vi "_script_update_doc_txt_stub.vi"() -> ()   [LabVIEW 2014]
uses:
  JKI State Machine++.lvlib
panel:
  out "States":string
  out "appended array":path[](array[path])
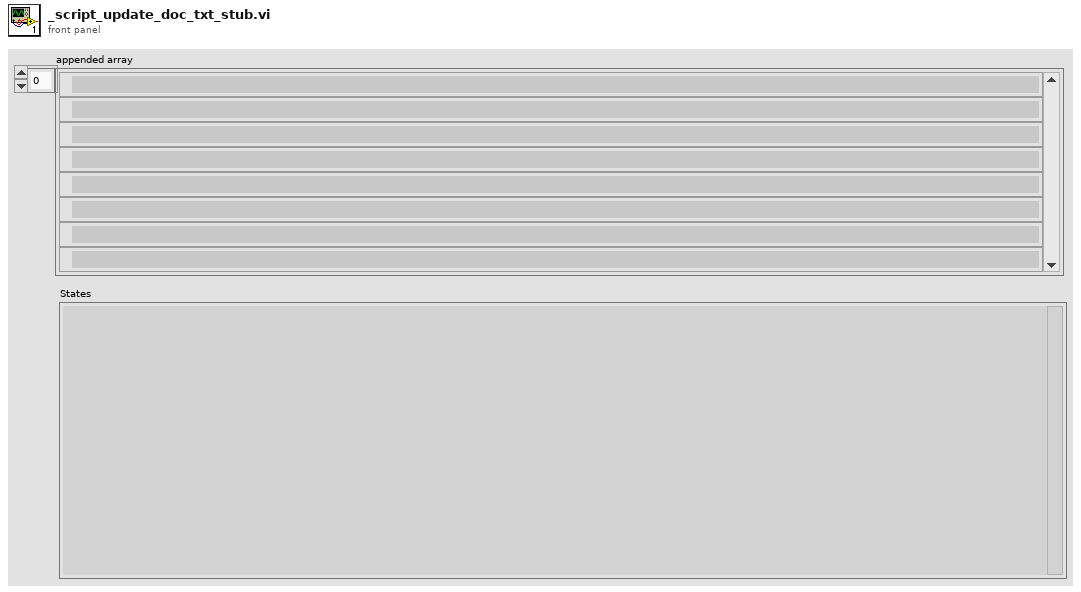
[diagram p1: front panel]
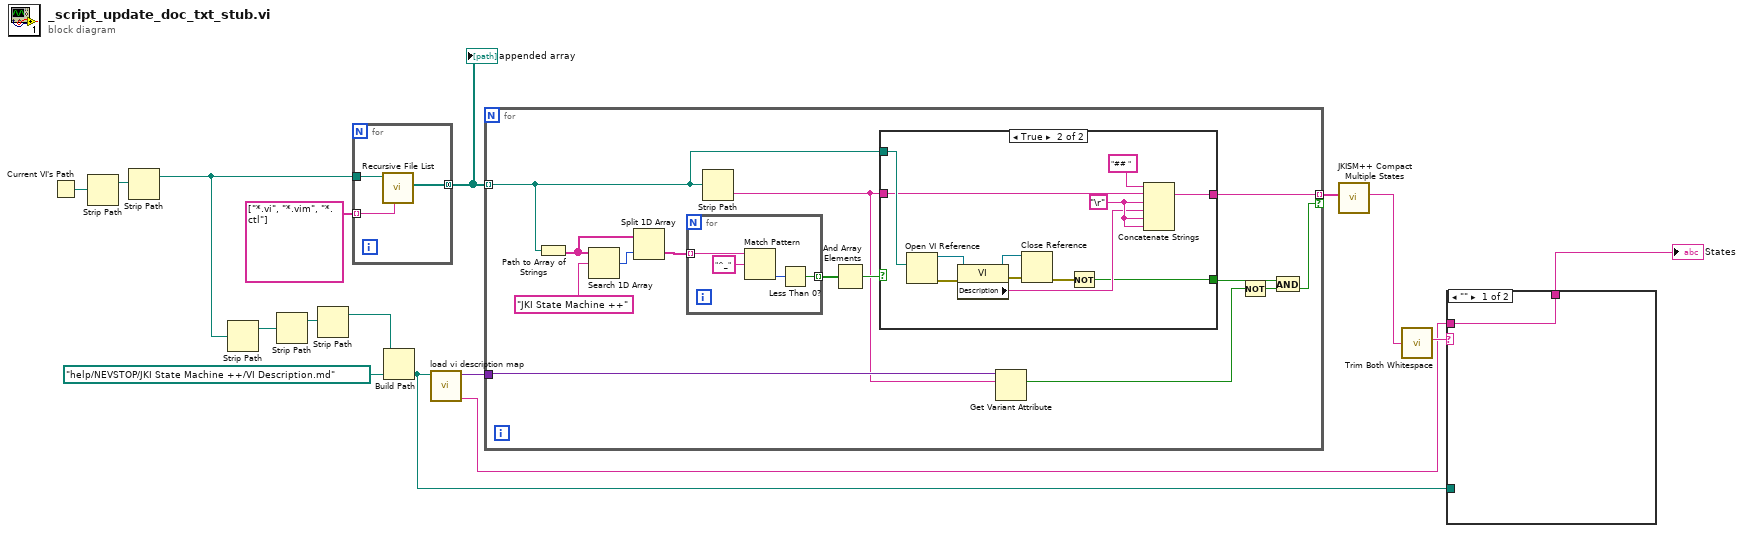
[diagram p0: block diagram]
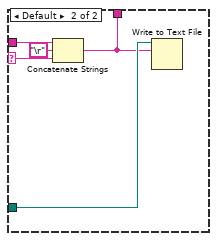
[diagram p2: hidden frame]
diagram:
  n1 = Current VI's Path() -> (path=w16:path)
  n2 = Strip Path(path=w16) -> (stripped path=w15:path)  [unwired: 1 out]
  n3 = Strip Path(path=w15) -> (stripped path=w6:path)  [unwired: 1 out]
  n4 = Strip Path(path=w6) -> (stripped path=w11:path)  [unwired: 1 out]
  n5 = Strip Path(path=w11) -> (stripped path=w12:path)  [unwired: 1 out]
  n6 = Strip Path(path=w12) -> (stripped path=w9:path)  [unwired: 1 out]
  n7 = for {
    tunnel: w6 -> [w19]
    tunnel: string[] ["*.vi", "*.vim", "*.ctl"] -> [w18] mode=indexing
    tunnel: [w17] -> w13 mode=concatenating
    n8 = call <vilib>:"Recursive File List.vi"("pattern"=w18, "Folder Path"=w19) -> ("All Files in Dir"=w17:path[])  [unwired: 5 in, 4 out]
  }
  "appended array" <- w13
  n9 = Build Path(base path=w9, name or relative path=path "help/NEVSTOP/JKI State Machine ++/VI Description.md" ("Path")) -> (appended path=w4:path)
  n10 = call "load vi description map.vi"("Path"=w4) -> ("text"=w2:string, "variant"=w7:variant)  [unwired: 9 in]
  n11 = for {
    tunnel: w13 -> [w31] mode=indexing
    tunnel: [w33] -> w8 mode=indexing if=w23
    tunnel: w7 -> [w25]
    n12 = Path to Array of Strings(0:w31) -> (2:w28:string[])  [unwired: 1 out]
    n13 = Search 1D Array(1D array=w28, element="JKI State Machine ++") -> (index of element=w29:i32)  [unwired: 1 in]
    n14 = Split 1D Array(array=w28, index=w29) -> (second subarray=w27:string[])  [unwired: 1 out]
    n15 = for {
      tunnel: [w35] -> w32 mode=indexing
      tunnel: w27 -> [w34] mode=indexing
      n16 = Match Pattern(string=w34, regular expression="^_") -> (offset past match=w36:i32)  [unwired: 1 in, 3 out]
      n17 = Less Than 0?(x=w36) -> (x < 0?=w35:bool)
    }
    n18 = Strip Path(path=w31) -> (name=w24:string)  [unwired: 1 out]
    n19 = And Array Elements(Boolean array=w32) -> (logical AND=w26:bool)
    n20 = case shown="True" w26 {
      tunnel: [_ w48] -> w33
      tunnel: w31 -> [_ w47]
      tunnel: [_ w39] -> w21
      tunnel: w24 -> [_ w38]
      frame False {
      }
      frame True {
        w42 = "\r"
        n21 = Open VI Reference(vi path=w47) -> (vi reference=w45:refnum<vi>, error out=w46:errorcluster)  [unwired: 5 in]
        n22 = property class="VI"(reference=w45, error in=w46) -> (reference out=w43:refnum<vi>, error out=w44:errorcluster, "Description"=w41:string)
        n23 = Close Reference(reference=w43, error in (no error)=w44) -> (error out=w40:errorcluster)
        n24 = Not(x=w40) -> (.not. x?=w39:bool)
        n25 = Concatenate Strings("## " ("string"), w38, w42, w41, w42, w42) -> (w48:string)
      }
    }
    n26 = Get Variant Attribute(Variant=w25, name=w24) -> (found=w22:bool)  [unwired: 2 in, 3 out]
    n27 = Not(x=w22) -> (.not. x?=w20:bool)
    n28 = And(x=w21, y=w20) -> (x .and. y?=w23:bool)
  }
  n29 = call "JKISM++ Compact Multiple States.vi"("States in Lines"=w8) -> ("States"=w5:string)  [unwired: 9 in]
  n30 = call "Trim Both Whitespace.vi"("string"=w5) -> ("trimmed string"=w3:string)  [unwired: 1 in]
  n31 = case shown="\"\"" w3 {
    selector: w3 -> [_ w53]
    tunnel: w4 -> [_ w54]
    tunnel: w2 -> [w50 w52]
    tunnel: [w50 w51] -> w1
    frame "" {
    }
    frame Default {
      n32 = Concatenate Strings(w52, "\r", w53) -> (w51:string)
      n33 = Write to Text File(file (use dialog)=w54, text=w51) -> ()  [unwired: 2 in, 3 out]
    }
  }
  "States" <- w1
